vi "WriteReadSPIforAD5781.vi"(0 "FPGA VI Reference Out 2":T3, 2 "DAC 18Bit Data":u32=16 format="%024b", 7 "SPI - AD5781 Setup":T2={"Port"=0, "Configuration Cluster"={"CS"=1, "Clock Rate (Hz)"=50000.0, "Clock Mode"=2, "CS Active State"=FALSE}, "Hardware Pins"={"RESET"=TRUE, "LDAC"=FALSE, "CLR"=TRUE}, "Total Bits"=8} {"Configuration Cluster"."CS" items=["0"=1, "1"=2, "2"=4, "3"=8, "4"=16, "5"=32, "6"=64, "7"=128]; "Configuration Cluster"."Clock Mode" items=["0", "1", "2", "3"]}, 11 "error in":errorcluster, 13 "register prefix":u8=16 format="%04b", 14 "2-Bit Suffix":u8 format="%02b") -> (4 "FPGA VI Reference Out":T3, 8 "Read Data":u8[](array[numeric]) format="%08b", 15 "error out":errorcluster)   [LabVIEW 2014]
uses:
  Host API/Controls/SPI Configuration Cluster.ctl
  Host API/Controls/FPGA Reference.ctl
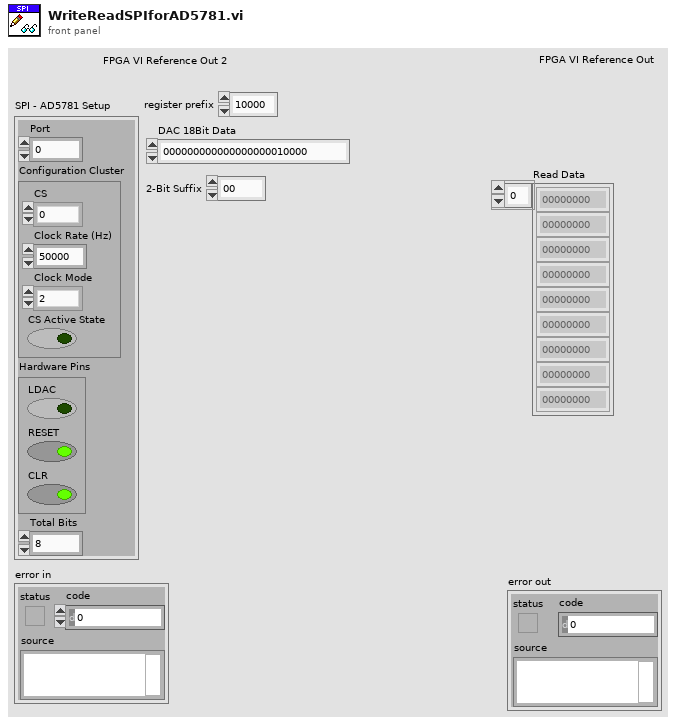
[diagram p1: front panel]
types:
  T1 = typedef "SPI Configuration Cluster.ctl" = cluster{"CS":u8, "Clock Rate (Hz)":dbl, "Clock Mode":u8, "CS Active State":bool}
  T2 = cluster{"Port":i8, "Configuration Cluster":T1, "Hardware Pins":cluster{"RESET":bool, "LDAC":bool, "CLR":bool}, "Total Bits":u16}
  T3 = typedef "FPGA Reference.ctl" = refnum<k20>
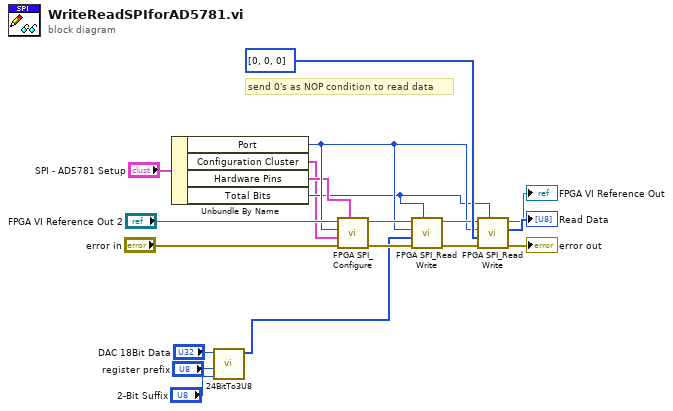
[diagram p0: block diagram]
diagram:
  # "send 0's as NOP condition to read data"
  n1 = Unbundle By Name("SPI - AD5781 Setup") -> ("Port"=w8:i8, "Configuration Cluster"=w5:T1, "Hardware Pins"=w7:cluster{"RESET":bool, "LDAC":bool, "CLR":bool}, "Total Bits"=w6:u16)
  n2 = call "24BitTo3U8.vi"("2-Bit Suffix"="2-Bit Suffix", "4-Bit Prefix"="register prefix", "18-Bit"="DAC 18Bit Data") -> ("3 U8"=w3:u8[])  [unwired: 8 in]
  n3 = call "FPGA SPI_Configure.vi"("Hardware Pins"=w7, "error in"="error in", "Configuration Cluster"=w5, "Port"=w8, "FPGA Interface"="FPGA VI Reference Out 2") -> ("error out"=w18:errorcluster, "FPGA VI Reference Out"=w19:refnum<k20>)  [unwired: 5 out]
  n4 = call "FPGA SPI_Read Write.vi"("Total Bits"=w6, "error in"=w18, "Write Data"=w3, "Port"=w8, "FPGA Interface"=w19) -> ("error out"=w14:errorcluster, "FPGA VI Reference Out"=w15:refnum<k20>)  [unwired: 5 out]
  n5 = call "FPGA SPI_Read Write.vi"("Total Bits"=w6, "error in"=w14, "Write Data"=u8[] [0, 0, 0], "Port"=w8, "FPGA Interface"=w15) -> ("error out"=→"error out":errorcluster, "Read Data"=→"Read Data":u8[], "FPGA VI Reference Out"=→"FPGA VI Reference Out":refnum<k20>)  [unwired: 4 out]
